vi "I-SRC Test Communications.vi"(8 "error in (no error)":errorcluster, 11 "VISA resource name in":refnum<visa-resource-name>) -> (0 "error out":errorcluster, 3 "VISA resource name out":refnum<visa-resource-name>)   [LabVIEW 2016, in "Hall Effect Library.lvlib"]
uses:
  Hall Effect Library.lvlib
  Global Variables/Instruments.vi
  I-SRC Test Communications (622x).vi
  I-SRC Test Communications (26XX).vi
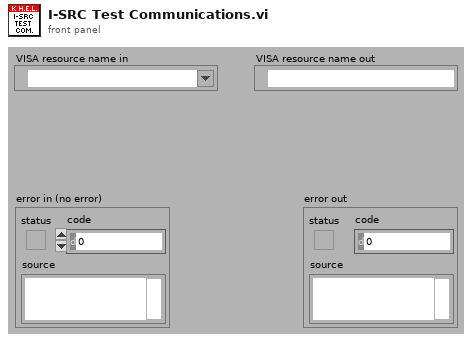
[diagram p1: front panel]
types:
  T1 = typedef "Hall Effect Library.lvlib/I-Sources.ctl" = enum16{"622X", "26XX"}
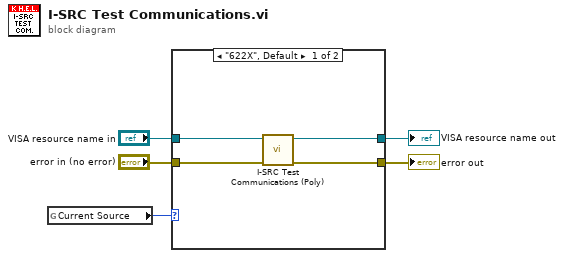
[diagram p0: block diagram]
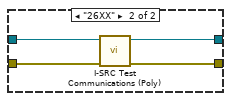
[diagram p2: hidden frame]
diagram:
  n1 = global read "Instruments.vi" "Current Source"() -> (w5:T1)
  n2 = case shown="\"622X\", Default" w5 {
    tunnel: "VISA resource name in" -> [w9 w13]
    tunnel: [w8 w12] -> w4
    tunnel: [w7 w11] -> w3
    tunnel: "error in (no error)" -> [w6 w10]
    frame "622X", Default {
      n3 = call-poly "I-SRC Test Communications (Poly).vi"("error in (no error)"=w6, "VISA resource name in"=w9) -> ("error out"=w7:errorcluster, "VISA resource name out"=w8:refnum<visa-resource-name>)  [unwired: 8 out]
    }
    frame "26XX" {
      n4 = call-poly "I-SRC Test Communications (Poly).vi"("error in (no error)"=w10, "VISA resource name in"=w13) -> ("error out"=w11:errorcluster, "VISA resource name out"=w12:refnum<visa-resource-name>)  [unwired: 8 out]
    }
  }
  "error out" <- w3
  "VISA resource name out" <- w4
